vi "Solartron 1260 multifile freq scan feb 15.vi"() -> ()   [LabVIEW 2014]
doc: "This VI configures and reads back a single measurement. \n\nNote:\nYou might need to extend the timeout set in the Wait Conditions subVI."
uses:
  <vilib>/Analysis/baseanly.llb/Mean (DBL).vi
  <vilib>/Utility/file.llb/Write To Spreadsheet File (string).vi
  <instrlib>/Solartron 1260/Solartron 1260.lvlib
  <vilib>/Analysis/NI_AALBase.lvlib
panel:
  out "File path":path
  out "XY Graph":cluster{dbl[], dbl[]}[](graph)
  in  "Variable, result source, citcuit 2":T1={"Variable (0:Frequency)"=enum."Frequency", "Result Source(0:Z1 = V1/I)"=enum."Z1 = V1/I", "Circuit (3:Parallel C, R)"=enum."Serial L, R", "Result Type(0: [Z, Theta] for: Z1 or Z2)"=enum."[Z, Theta]       for: Z1 or Z2", "DC Bias (V)"=0.0, "Amplitude (V)"=1.0} {"Amplitude (V)" min=0.0 max=3.0 format="%^.3e"; "DC Bias (V)" min=-42.0 max=42.0 format="%^.3e"}
  in  "measure spectra":bool
  out "Total scan time (hrs)":dbl
  out "Spectrum scan time (min)":dbl
  out "Freq. resolution (Hz)":dbl
  in  "Frequency options":T2={"End freq (Hz)"=0.0, "Start freq (Hz)"=0.0, "# of freq steps in each spectrum"=0.0, "# of steps to average"=3.0, "# of spectra to measure"=3.0} {"Start freq (Hz)" format="%#_8f"; "End freq (Hz)" format="%#_8f"}
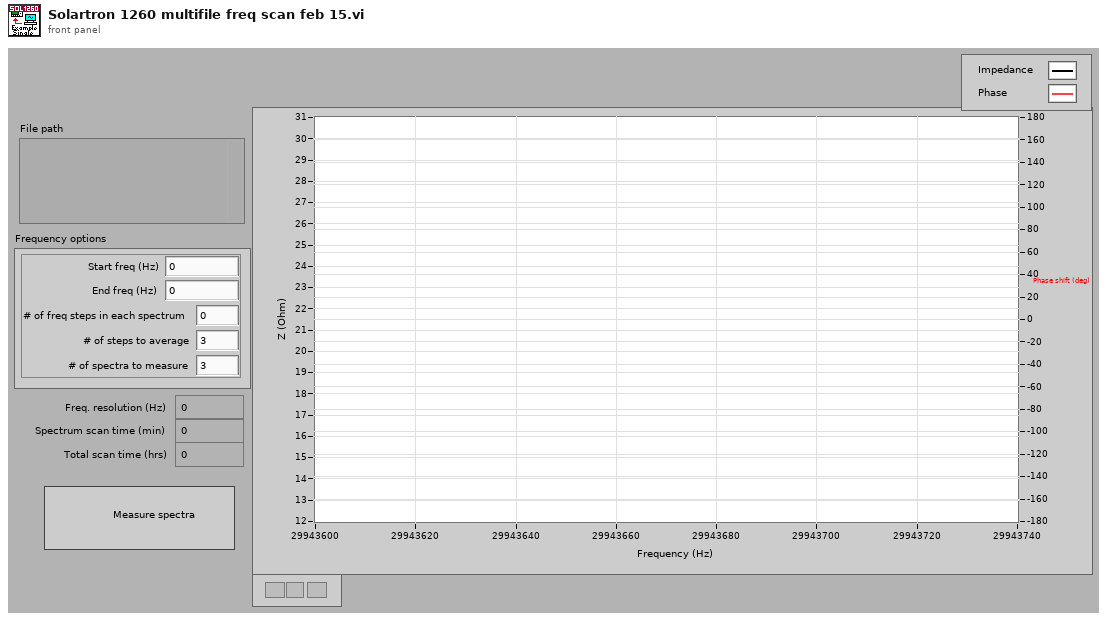
[diagram p1: front panel]
types:
  T1 = cluster{"Variable (0:Frequency)":enum16{"Frequency", "Amplitude", "Baise"}, "Result Source(0:Z1 = V1/I)":enum16{"Z1 = V1/I", "Y1 = I/V1", "Z2 = V2/I", "Y2 = I/V2", "Function (  )", "V1", "V2", "V1/V2", "V2/V1", " I"}, "Circuit (3:Parallel C, R)":enum16{"Serial L, R", "Serial C, R", "Parallel L, R", "Parallel C, R", "Auto"}, "Result Type(0: [Z, Theta] for: Z1 or Z2)":enum16{"[Z, Theta]       for: Z1 or Z2", "[Y, Theta]       for: Y1 or Y2", "[r, Theta]        for: Fnc( ), V1, V2, V1/V2, V2/V1 or I", "[r(dB), Theta]  for: Fnc( ), V1, V2, V1/V2 or V2/V1", "[r, t]                 for: Fnc( ), V1, V2, V1/V2 or V2/V1", "[r (dB), t]          for: Fnc( ), V1, V2, V1/V2 or V2/V1", "[L(or C), R]      for: Z1, Y1, Z2, Y2 or Fnc( )", "[L(or C), Q]      for: Z1, Y1, Z2, Y2 or Fnc( )", "[L(or C), D]      for: Z1, Y1, Z2, Y2 or Fnc( ) ", "[R, X]              for: Z1 or Z2", "[G, B]              for: Y1 or Y2", "[a, b]               for: Fnc( ), V1, V2, V1/V2, V2/V1 or I"}, "DC Bias (V)":dbl, "Amplitude (V)":dbl}
  T2 = cluster{"End freq (Hz)":dbl, "Start freq (Hz)":dbl, "# of freq steps in each spectrum":dbl, "# of steps to average":dbl, "# of spectra to measure":dbl}
  T3 = enum16{"Off", "All", "Fail", "Pass", "Dump", "Dump all", "Plotter"}
  T4 = enum16{"Z1 = V1/I", "Y1 = I/V1", "Z2 = V2/I", "Y2 = I/V2", "Function (  )", "V1", "V2", "V1/V2", "V2/V1", " I"}
  T5 = enum16{"Serial L, R", "Serial C, R", "Parallel L, R", "Parallel C, R", "Auto"}
  T6 = enum16{"[Z, Theta]       for: Z1 or Z2", "[Y, Theta]       for: Y1 or Y2", "[r, Theta]        for: Fnc( ), V1, V2, V1/V2, V2/V1 or I", "[r(dB), Theta]  for: Fnc( ), V1, V2, V1/V2 or V2/V1", "[r, t]                 for: Fnc( ), V1, V2, V1/V2 or V2/V1", "[r (dB), t]          for: Fnc( ), V1, V2, V1/V2 or V2/V1", "[L(or C), R]      for: Z1, Y1, Z2, Y2 or Fnc( )", "[L(or C), Q]      for: Z1, Y1, Z2, Y2 or Fnc( )", "[L(or C), D]      for: Z1, Y1, Z2, Y2 or Fnc( ) ", "[R, X]              for: Z1 or Z2", "[G, B]              for: Y1 or Y2", "[a, b]               for: Fnc( ), V1, V2, V1/V2, V2/V1 or I"}
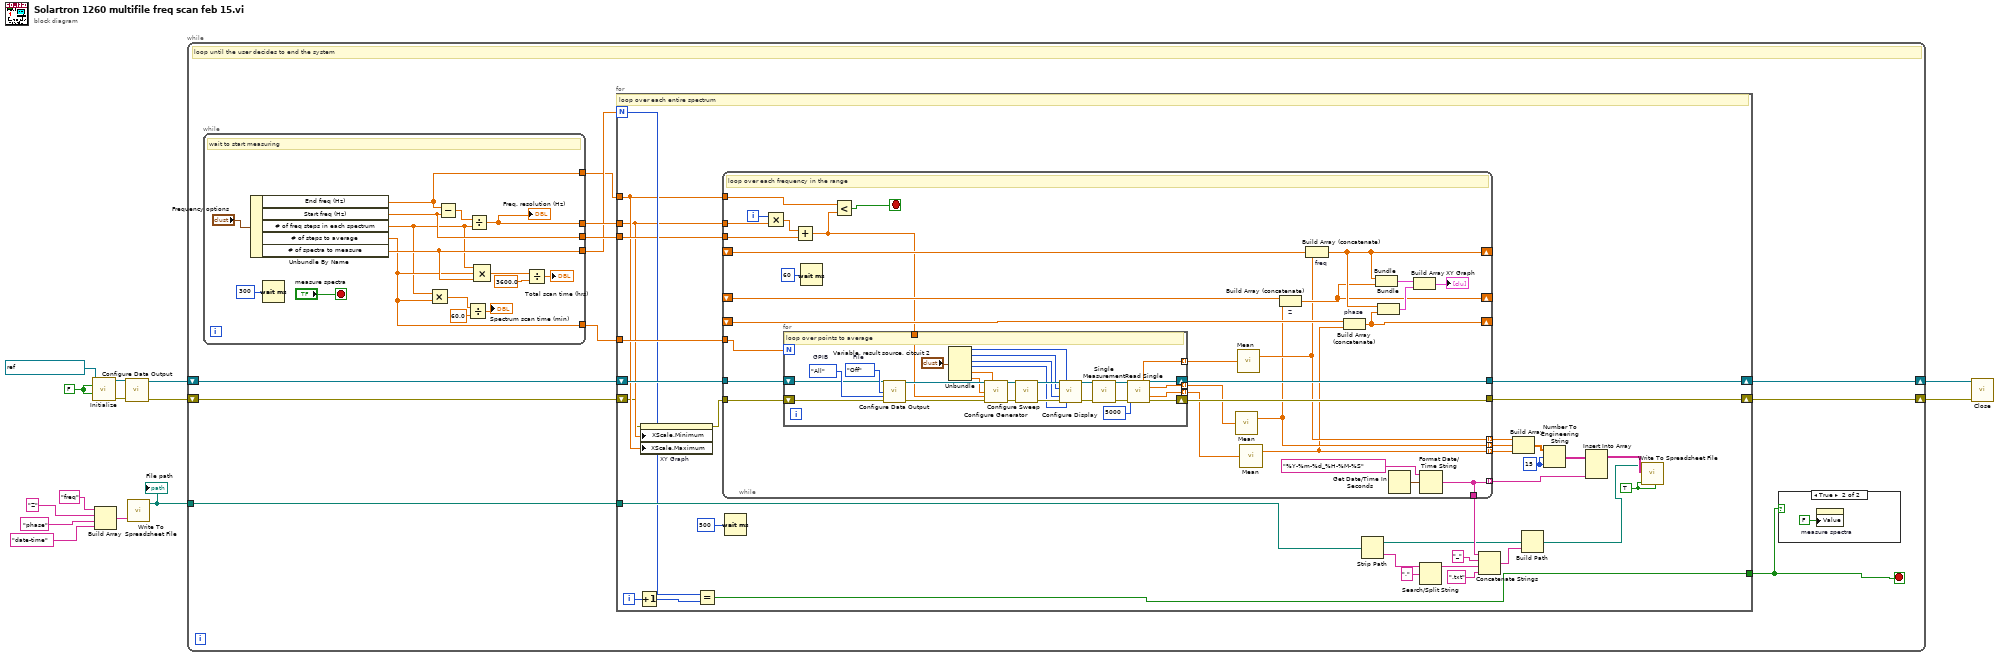
[diagram p0: block diagram]
diagram:
  w12 = FALSE ("ID Query (T: Check)")
  n1 = call <instrlib>:"Initialize.vi"("VISA resource name"=refnum<visa-resource-name> "GPIB2::4::INSTR", "ID Query (T: Check)"=w12, "Reset (T: Reset)"=w12) -> ("VISA resource name out"=w9:refnum<visa-resource-name>, "error out"=w10:errorcluster)  [unwired: 11 in]
  n2 = Build Array("freq", "Z", "phase", "date-time") -> (w3:string[])
  n3 = call <instrlib>:"Configure Data Output.vi"("VISA resource name"=w9, "error in (no error)"=w10) -> ("VISA resource name out"=w8:refnum<visa-resource-name>, "error out"=w7:errorcluster)  [unwired: 12 in]
  n4 = call-poly <vilib>:"Write To Spreadsheet File.vi"("1D data"=w3) -> ("new file path (Not A Path if cancelled)"=w2:path)  [unwired: 7 in]
  "File path" <- w2
  n5 = while {
    shift-right: [w24] -> w13
    shift-left: w8 -> [w23]
    shift-right: [w25] -> w14
    shift-left: w7 -> [w22]
    tunnel: w2 -> [w18]
    stop <- w15 stop-if-true
    # "loop until the user decides to end the system"
    n6 = while {
      tunnel: [w41] -> w21
      tunnel: [w29] -> w20
      tunnel: [w38] -> w19
      tunnel: [w33] -> w17
      tunnel: [w35] -> w16
      stop <- "measure spectra" stop-if-true
      # "wait to start measuring"
      n7 = Unbundle By Name("Frequency options") -> ("End freq (Hz)"=w35:dbl, "Start freq (Hz)"=w41:dbl, "# of freq steps in each spectrum"=w28:dbl, "# of steps to average"=w29:dbl, "# of spectra to measure"=w33:dbl)
      n8 = Wait (ms)(milliseconds to wait=300) -> ()  [unwired: 1 out]
      n9 = Multiply(x=w28, y=w29) -> (x*y=w30:dbl)
      n10 = Subtract(x=w35, y=w41) -> (x-y=w42:dbl)
      n11 = Divide(x=w30, y=60.0) -> (x/y=→"Spectrum scan time (min)":dbl)
      n12 = Divide(x=w42, y=w28) -> (x/y=w38:dbl)
      "Freq. resolution (Hz)" <- w38
      n13 = Compound Arithmetic op=MULTIPLY(w28, w29, w33) -> (w27:dbl)
      n14 = Divide(x=w27, y=3600.0) -> (x/y=→"Total scan time (hrs)":dbl)
    }
    n15 = for {
      N: w17 -> [w51]
      tunnel: w21 -> [w47]
      tunnel: w16 -> [w46]
      tunnel: w20 -> [w72]
      tunnel: w19 -> [w45]
      tunnel: w18 -> [w61]
      shift-right: [w74] -> w24
      shift-left: w23 -> [w73]
      shift-right: [w75] -> w25
      shift-left: w22 -> [w43]
      tunnel: [w50] -> w15
      i -> [w49]
      w70 = TRUE ("append to file? (new file:F)")
      w71 = i16 15 ("precision (6)")
      # "loop over each entire spectrum"
      n16 = Increment(x=w49) -> (x+1=w48:i32)
      n17 = property on="XY Graph" class="XYGraph (strict)"(error in=w43, "XScale.Minimum"=w45, "XScale.Maximum"=w46) -> (error out=w44:errorcluster)  [unwired: 1 in, 1 out]
      n18 = Equal?(x=w51, y=w48) -> (x = y?=w50:bool)
      n19 = while {
        tunnel: [w100] -> w75
        tunnel: [w99] -> w74
        tunnel: w73 -> [w102]
        tunnel: w44 -> [w101]
        tunnel: w47 -> [w103]
        shift-right: [w90] -> _
        shift-left: _ -> [w98]
        shift-right: [w89] -> _
        shift-left: _ -> [w97]
        tunnel: w45 -> [w96]
        shift-right: [w92] -> _
        shift-left: _ -> [w93]
        tunnel: [w80] -> w69 mode=indexing
        tunnel: [w78] -> w67 mode=indexing
        tunnel: [w76] -> w68 mode=indexing
        tunnel: w46 -> [w87]
        tunnel: w72 -> [w88]
        tunnel: [w84] -> w65 mode=indexing
        tunnel: [w84] -> w54
        i -> [w105]
        stop <- w82 stop-if-true
        # "loop over each frequency in the range"
        n20 = Multiply(x=w105, y=w96) -> (x*y=w104:dbl)
        n21 = Add(x=w104, y=w103) -> (x+y=w86:dbl)
        n22 = for {
          N: w88 -> [_]
          tunnel: [w112] -> w81 mode=indexing
          tunnel: [w111] -> w79 mode=indexing
          tunnel: [w110] -> w77 mode=indexing
          tunnel: w86 -> [w109]
          shift-right: [w118] -> w99
          shift-left: w102 -> [w121]
          shift-right: [w119] -> w100
          shift-left: w101 -> [w120]
          w123 = T3."All"  # GPIB
          w124 = enum16{"Off", "All", "Fail", "Pass"}."Off"  # File
          # "loop over points to average"
          n23 = call <instrlib>:"Configure Data Output.vi"("VISA resource name"=w121, "File (1:All)"=w124, "GPIB (1:All)"=w123, "error in (no error)"=w120) -> ("VISA resource name out"=w133:refnum<visa-resource-name>, "error out"=w134:errorcluster)  [unwired: 10 in]
          n24 = Unbundle("Variable, result source, citcuit 2") -> ("Variable (0:Frequency)"=w116:enum16{"Frequency", "Amplitude", "Baise"}, "Result Source(0:Z1 = V1/I)"=w114:T4, "Circuit (3:Parallel C, R)"=w115:T5, "Result Type(0: [Z, Theta] for: Z1 or Z2)"=w113:T6, "DC Bias (V)"=w108:dbl, "Amplitude (V)"=w107:dbl)
          n25 = call <instrlib>:"Configure Generator.vi"("VISA resource name"=w133, "Voltage Bias(0.0 V)"=w108, "Voltage Amplitude(1.0 V)"=w107, "Frequency(1.0 Hz)"=w109, "error in (no error)"=w134) -> ("VISA resource name out"=w132:refnum<visa-resource-name>, "error out"=w131:errorcluster)  [unwired: 9 in]
          n26 = call <instrlib>:"Configure Sweep.vi"("VISA resource name"=w132, "error in (no error)"=w131) -> ("VISA resource name out"=w129:refnum<visa-resource-name>, "error out"=w130:errorcluster)  [unwired: 12 in]
          n27 = call <instrlib>:"Configure Display.vi"("VISA resource name"=w129, "Variable (0:Frequency)"=w116, "Result Source(0:Z1 = V1/I)"=w114, "Circuit (3:Parallel C, R)"=w115, "error in (no error)"=w130, "Result Type(0: [Z, Theta] for: Z1 or Z2)"=w113) -> ("VISA resource name out"=w128:refnum<visa-resource-name>, "error out"=w127:errorcluster)  [unwired: 8 in]
          n28 = call <instrlib>:"Single Measurement.vi"("VISA resource name"=w128, "error in (no error)"=w127) -> ("VISA resource name out"=w125:refnum<visa-resource-name>, "error out"=w126:errorcluster)  [unwired: 12 in]
          n29 = call <instrlib>:"Read Single.vi"("VISA resource name"=w125, "timeout ms (5000)"=u32 5000, "error in (no error)"=w126) -> ("Variable"=w112:dbl, "VISA resource name out"=w118:refnum<visa-resource-name>, "Parameter 1"=w111:dbl, "Parameter2"=w110:dbl, "error out"=w119:errorcluster)  [unwired: 6 in, 2 out]
        }
        n30 = Wait (ms)(milliseconds to wait=u32 60) -> ()  [unwired: 1 out]
        n31 = Less?(x=w87, y=w86) -> (x < y?=w82:bool)
        n32 = call-poly <vilib>:"Mean.vi"("X"=w79) -> ("mean"=w78:dbl)  [unwired: 1 out]
        n33 = call-poly <vilib>:"Mean.vi"("X"=w81) -> ("mean"=w80:dbl)  [unwired: 1 out]
        n34 = call-poly <vilib>:"Mean.vi"("X"=w77) -> ("mean"=w76:dbl)  [unwired: 1 out]
        n35 = Build Array (concatenate) "Z"(w97, w78) -> (w89:dbl[])
        n36 = Build Array (concatenate) "freq"(w98, w80) -> (w90:dbl[])
        n37 = Build Array (concatenate) "phase"(w93, w76) -> (w92:dbl[])
        n38 = Bundle(w90, w89) -> (w95:cluster{dbl[], dbl[]})  [unwired: 1 in]
        n39 = Bundle(w90, w92) -> (w94:cluster{dbl[], dbl[]})  [unwired: 1 in]
        n40 = Get Date/Time In Seconds() -> (seconds since 1Jan1904=w85:timestamp)
        n41 = Build Array(w95, w94) -> (→"XY Graph":cluster{dbl[], dbl[]}[])
        n42 = Format Date/Time String(time format string (%c)="%Y-%m-%d_%H-%M-%S", seconds (now)=w85) -> (date/time string=w84:string)  [unwired: 1 in]
      }
      n43 = Wait (ms)(milliseconds to wait=500) -> ()  [unwired: 1 out]
      n44 = Strip Path(path=w61) -> (stripped path=w53:path, name=w56:string)
      n45 = Search/Split String(string=w56, search string/char (-)=".") -> (substring before match=w57:string)  [unwired: 1 in, 2 out]
      n46 = Concatenate Strings(w54, "_" ("string"), w57, ".txt" ("string")) -> (w59:string)
      n47 = Build Array(w69, w67, w68) -> (w64:dbl[][])
      n48 = Build Path(base path=w53, name or relative path=w59) -> (appended path=w52:path)
      n49 = Number To Engineering String(2:w71, 3:w71, 4:w64) -> (0:w66:string[][])  [unwired: 1 in]
      n50 = Insert Into Array(array=w66, new element=w65) -> (w63:string[][])  [unwired: 2 in]
      n51 = call-poly <vilib>:"Write To Spreadsheet File.vi"("transpose? (no:F)"=w70, "append to file? (new file:F)"=w70, "2D data"=w63, "file path (dialog if empty)"=w52) -> ()  [unwired: 4 in, 1 out]
    }
    n52 = case shown="True" w15 {
      frame False {
      }
      frame True {
        n53 = property on="measure spectra" class="Bool (strict)"("Value"=FALSE ("measure spectrum")) -> ()  [unwired: 2 in, 2 out]
      }
    }
  }
  n54 = call <instrlib>:"Close.vi"("VISA resource name"=w13, "error in (no error)"=w14) -> ()  [unwired: 13 in, 1 out]
